vi "BoxSimShoot.vi"() -> ()   [LabVIEW 2023]
uses:
  BoxSystem/BoxStatesEnum.ctl
  BoxSystem/BoxNoteState.ctl
  <vilib>/Rock Robotics/WPI/ThirdParty/JAS_Junk/TrajLib/Enum/DCMOTOR_TYPES_ENUM.ctl
  <vilib>/Rock Robotics/WPI/ThirdParty/JAS_Junk/TrajLib/VI/Util_GetTime_U32.vi
  <vilib>/Rock Robotics/WPI/ThirdParty/JAS_Junk/TrajLib/VI/DigSeqLogic_Edge_On.vi
  <vilib>/Rock Robotics/WPI/ThirdParty/JAS_Junk/TrajLib/VI/BoolCmd_Send_Internal.vi
  <vilib>/Rock Robotics/WPI/ThirdParty/JAS_Junk/TrajLib/SlewRateLimiter_New.vi
  <vilib>/Rock Robotics/WPI/ThirdParty/JAS_Junk/TrajLib/SlewRateLimiter_Reset.vi
  <vilib>/Rock Robotics/WPI/ThirdParty/JAS_Junk/TrajLib/SlewRateLimiter_Calculate.vi
  <vilib>/Rock Robotics/WPI/ThirdParty/JAS_Junk/TrajLib/SlewRateLimiter_SetRate.vi
  <vilib>/Rock Robotics/WPI/ThirdParty/JAS_Junk/TrajLib/VI/BoolCmd_ObtainQueue.vi
  <vilib>/Rock Robotics/WPI/ThirdParty/JAS_Junk/TrajLib/VI/Util_GetTime_U64.vi
  <vilib>/Rock Robotics/WPI/ThirdParty/JAS_Junk/TrajLib/Trajectory_Library.lvlib
panel:
  out "Intake Control":T1(graph)
  in  "Cancel":bool
  in  "Amp":bool
  in  "Source":bool
  in  "Intake":bool
  in  "Shoot":bool
  out "Box Note State":T2
  out "StateMachineState":T3=enum."initilization"
  in  "Intake Sensor\nOff=BeamBroken":bool
  in  "Shoot Sensor\nOff=BeamBroken":bool
  out "Velocity_Filtered RPM R":dbl format="%13.1f"
  out "Velocity_Filtered RPM":dbl format="%13.1f"
  out "Motor DmdR (CO)":dbl format="%10.3f"
  out "AtSetpoint R":bool
  out "FeedForward R":dbl
  out "VelocityR_RPM":dbl format="%13.1f"
  in  "Auto R":bool=TRUE
  out "ShooterR Control":T4(graph)
  out "Battery Voltage":dbl format="%10.1f"
  out "ShooterL Control":T1(graph)
  in  "Auto":bool=TRUE
  out "VelocityL_RPM":dbl format="%13.1f"
  out "FeedForward":dbl
  out "AtSetpointL":bool
  out "MotorL Dmd (CO)":dbl format="%10.3f"
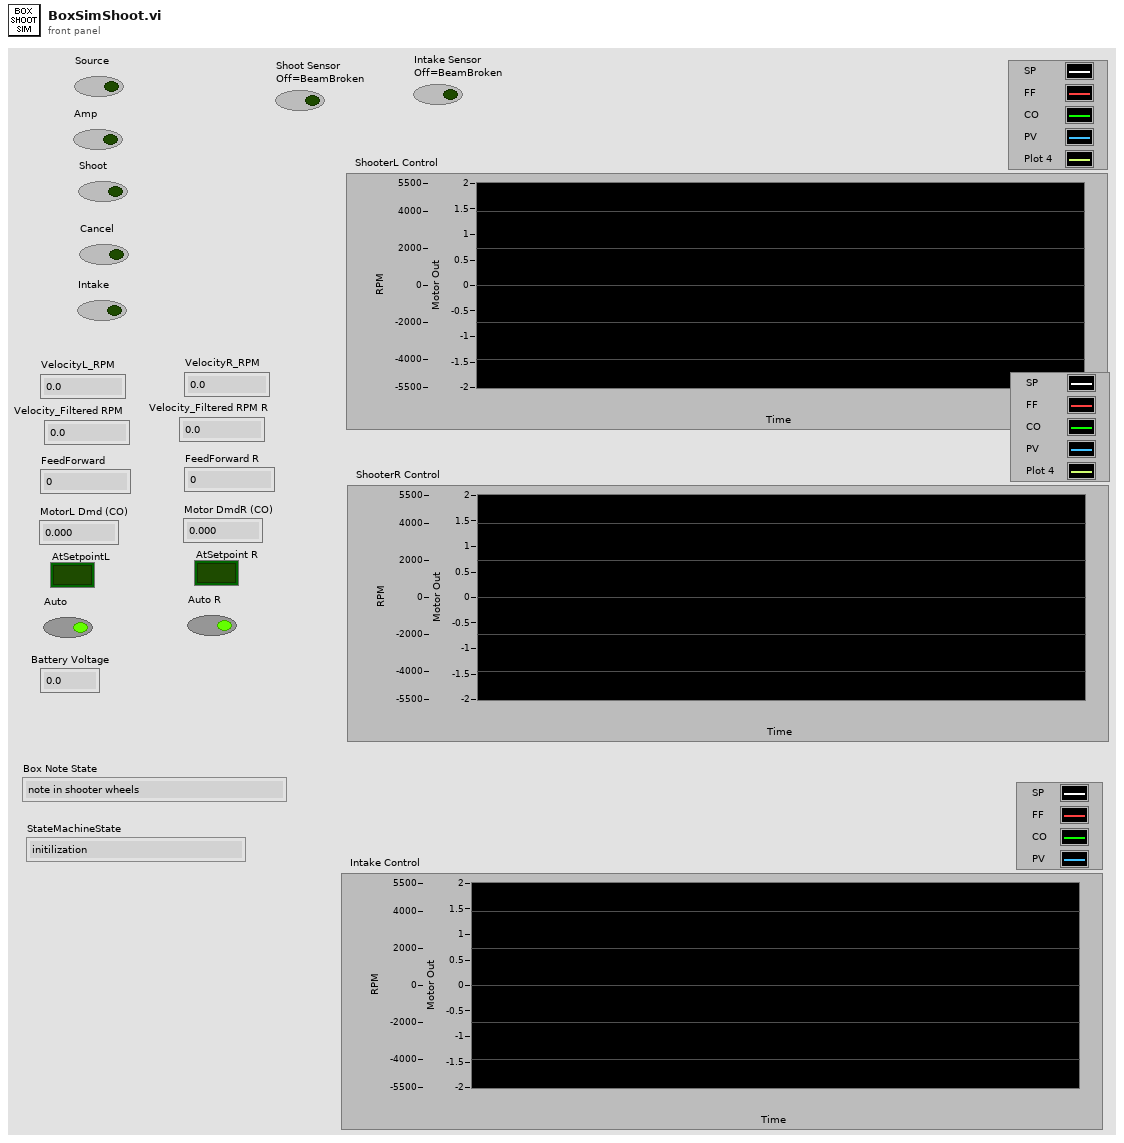
[diagram p1: front panel]
types:
  T1 = cluster{"ShootL SP":dbl, "ShootL FF":dbl, "ShootLOut":dbl, "Velocity_RPM":dbl, "ShootL Filt RPM":dbl}
  T2 = typedef "BoxNoteState.ctl" = enum16{"note in shooter wheels", "misaligned note", "no note", "have note"}
  T3 = typedef "BoxStatesEnum.ctl" = enum16{"get input", "start shoot wheels", "up to speed?", "run intake", "have ring?", "stop intake and shooter", "start intake", "pick up ring or  _ sec?", "stop intake", "start source  intake", "pick up note?", "stop intake shooter", "shoot amp", "used note?", "stop amp intake", "initilization"}
  T4 = cluster{"ShootR SP":dbl, "ShootR FF":dbl, "ShootROut":dbl, "Velocity_RPM":dbl, "ShootR Filt RPM":dbl}
  T5 = cluster{"Shoot Sensor":bool, "Intake Sensor":bool, "ShootLSpeed":dbl, "ShootRSpeed":dbl, "IntakeSpeed":dbl}
  T6 = typedef "Trajectory_Library.lvlib/DCMOTOR_TYPES_ENUM.ctl" = enum16{"CIM", "AndyMark 9015", "Andy Mark RS 775 125", "Bag", "BaneBots RS 550", "BaneBots RS 775", "Falcon 500", "Mini CIM", "NEO", "NEO 550", "Romi BuiltIn", "Vex 775 Pro", "Snow Blower AM 2235A", "Bosch Seat AM 3493"}
  T7 = cluster{"ShootLOnTarg":bool, "ShootROnTarg":bool, "StateMachineState":T3, "Box Note State":T2, "ShootR SP":dbl, "ShootR FF":dbl, "ShootR Filt RPM":dbl, "ShootL SP":dbl, "ShootL FF":dbl, "ShootL Filt RPM":dbl}
  T8 = cluster{"ShootLOut":dbl, "ShootROut":dbl, "IntakeOut":dbl}
  T9 = typedef "Trajectory_Library.lvlib/LINEAR_SYSTEM_ID_FLYWHEEL_MODEL.ctl" = cluster{"DCMOTOR_TYPES":T6, "Num Motors":i32, "Gearing":dbl, "MOI kgm2":dbl}
  T10 = typedef "Trajectory_Library.lvlib/FLYWHEEL_SIM_SIMULATION_PARAMS.ctl" = cluster{"Vel Meas Std Dev Rad/Sec":dbl}
  T11 = cluster{dbl, dbl, "IntakeOut":dbl, "Velocity_RPM":dbl, "Velocity_RPM":dbl}
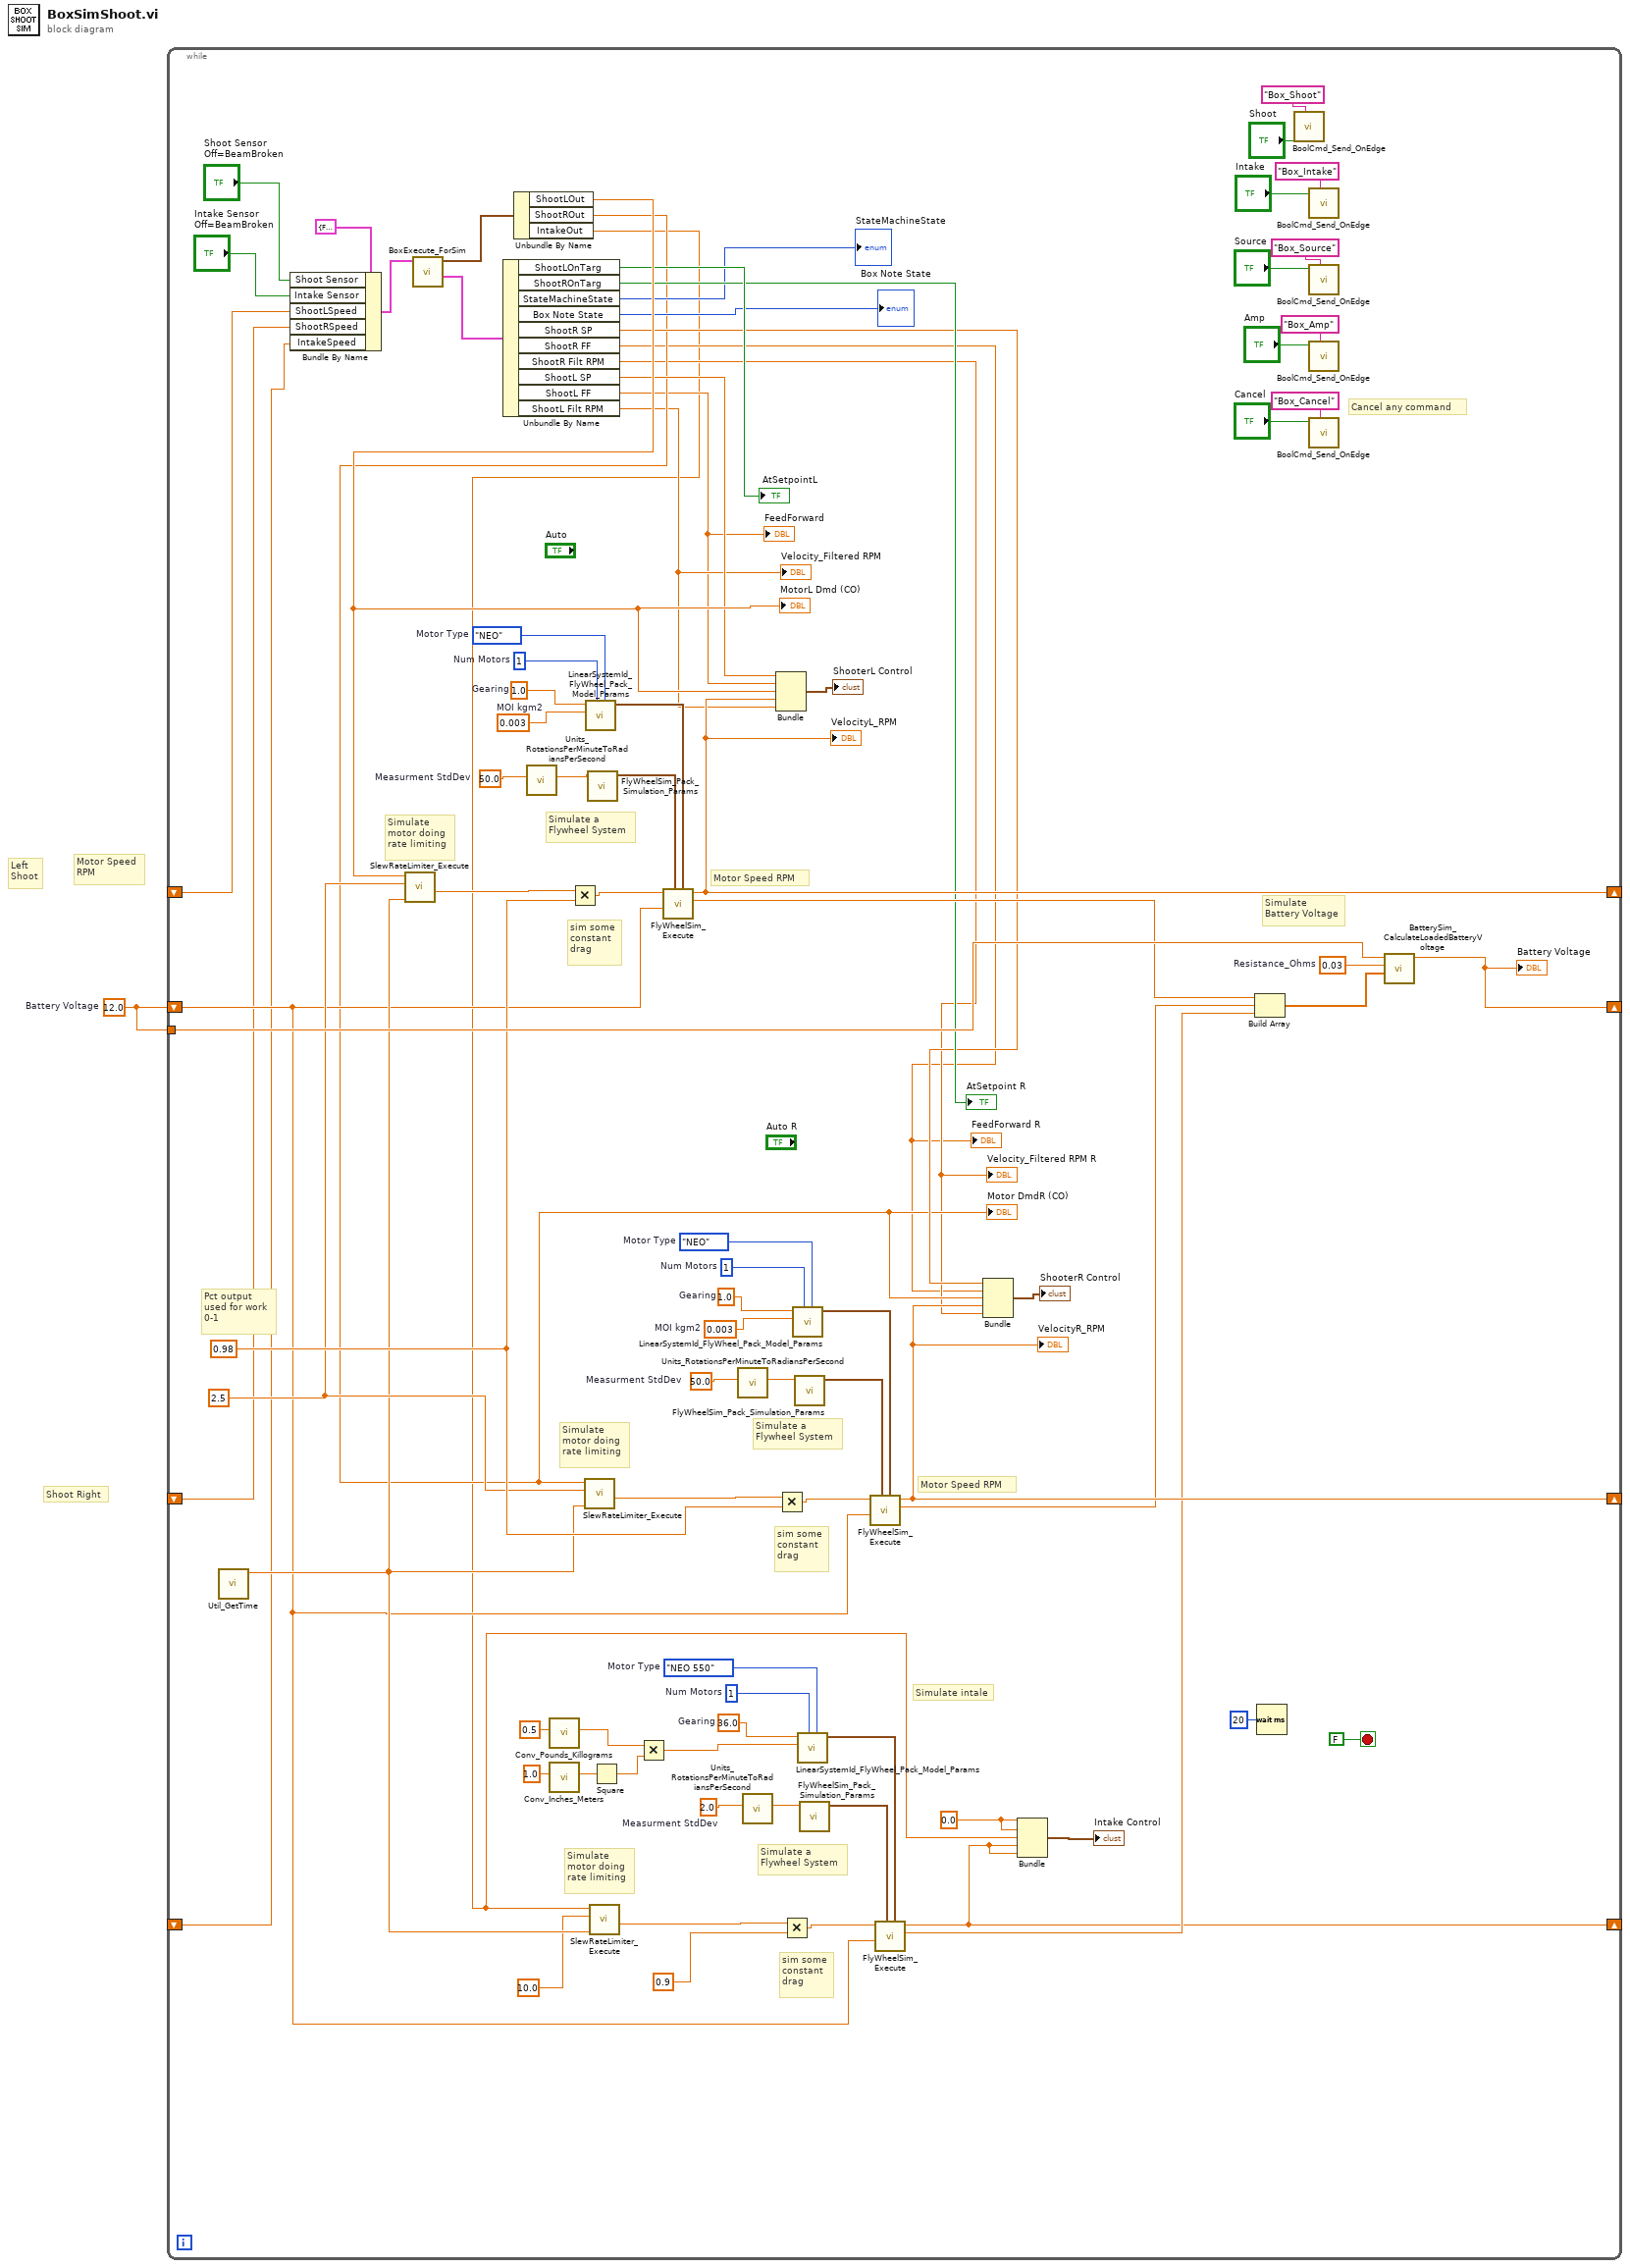
[diagram p0: block diagram]
diagram:
  w1 = 12.0  # Battery Voltage
  # "Shoot Right"
  # "Left\nShoot"
  # "Motor Speed\nRPM"
  n1 = while {
    shift-right: [w66] -> _
    shift-left: w1 -> [w38]
    shift-right: [w80] -> _
    shift-left: _ -> [w33]
    tunnel: w1 -> [w67]
    shift-right: [w69] -> _
    shift-left: _ -> [w32]
    shift-right: [w2] -> _
    shift-left: _ -> [w28]
    stop <- FALSE stop-if-true
    w4 = 0.0
    w48 = 2.0  # Measurment StdDev
    w50 = 36.0  # Gearing
    w51 = 1  # Num Motors
    w52 = DCMOTOR_TYPES_ENUM."NEO 550"  # Motor Type
    w58 = 50.0  # Measurment StdDev
    w61 = 2.5 ("y")
    w68 = 0.03  # Resistance_Ohms
    w59 = 50.0  # Measurment StdDev
    w70 = 1.0  # Gearing
    w71 = 0.003  # MOI kgm2
    w72 = 1  # Num Motors
    w73 = DCMOTOR_TYPES_ENUM."NEO"  # Motor Type
    w62 = 0.98 ("y")
    w87 = 1.0  # Gearing
    w88 = 0.003  # MOI kgm2
    w89 = 1  # Num Motors
    w90 = DCMOTOR_TYPES_ENUM."NEO"  # Motor Type
    # "Cancel any command"
    # "Simulate intale"
    # "Simulate\nmotor doing\nrate limiting"
    # "sim some\nconstant\ndrag"
    # "Simulate a \nFlywheel System"
    # "Pct output\nused for work\n0-1"
    # "Simulate\nmotor doing\nrate limiting"
    # "sim some\nconstant\ndrag"
    # "Motor Speed RPM"
    # "Simulate a \nFlywheel System"
    # "Simulate\nmotor doing\nrate limiting"
    # "sim some\nconstant\ndrag"
    # "Motor Speed RPM"
    # "Simulate\nBattery Voltage"
    # "Simulate a \nFlywheel System"
    n2 = call <vilib>:"Util_GetTime.vi"() -> ("FPGA_Time_Seconds"=w39:dbl)  [unwired: 9 in, 2 out]
    n3 = Bundle By Name(cluster=T5 {"Shoot Sensor"=FALSE, "Intake Sensor"=FALSE, "ShootLSpeed"=0.0, "ShootRSpeed"=0.0, "IntakeSpeed"=0.0} ("Inputs"), "Shoot Sensor"="Shoot Sensor\nOff=BeamBroken", "Intake Sensor"="Intake Sensor\nOff=BeamBroken", "ShootLSpeed"=w33, "ShootRSpeed"=w32, "IntakeSpeed"=w28) -> (w34:T5)
    n4 = call "BoxExecute_ForSim.vi"("Inputs"=w34) -> ("OtherOutputs"=w36:T7, "Outputs"=w37:T8)  [unwired: 9 in]
    n5 = Unbundle By Name(w36) -> ("ShootLOnTarg"=→"AtSetpointL":bool, "ShootROnTarg"=→"AtSetpoint R":bool, "StateMachineState"=→"StateMachineState":T3, "Box Note State"=→"Box Note State":T2, "ShootR SP"=w21:dbl, "ShootR FF"=w18:dbl, "ShootR Filt RPM"=w19:dbl, "ShootL SP"=w22:dbl, "ShootL FF"=w16:dbl, "ShootL Filt RPM"=w17:dbl)
    "FeedForward" <- w16
    "Velocity_Filtered RPM" <- w17
    "FeedForward R" <- w18
    "Velocity_Filtered RPM R" <- w19
    n6 = Unbundle By Name(w37) -> ("ShootLOut"=w31:dbl, "ShootROut"=w20:dbl, "IntakeOut"=w3:dbl)
    "MotorL Dmd (CO)" <- w31
    "Motor DmdR (CO)" <- w20
    n7 = call <vilib>:"SlewRateLimiter_Execute.vi"("Time"=w39, "PositiveRate"=w61, "Input"=w31) -> ("Output"=w79:dbl)  [unwired: 7 in, 1 out]
    n8 = call <vilib>:"Units_RotationsPerMinuteToRadiansPerSecond.vi"("RotationsPerMinute"=w58) -> ("RadiansPerSecond"=w57:dbl)  [unwired: 10 in]
    n9 = call <vilib>:"Conv_Pounds_Killograms.vi"("Pounds"=0.5) -> ("Killograms"=w45:dbl)  [unwired: 10 in]
    n10 = call <vilib>:"Conv_Inches_Meters.vi"("INCH"=1.0) -> ("Meters"=w47:dbl)  [unwired: 10 in]
    n11 = Multiply(x=w79, y=w62) -> (x*y=w82:dbl)
    n12 = call <vilib>:"SlewRateLimiter_Execute.vi"("Time"=w39, "PositiveRate"=w61, "Input"=w20) -> ("Output"=w78:dbl)  [unwired: 7 in, 1 out]
    n13 = call <vilib>:"LinearSystemId_FlyWheel_Pack_Model_Params.vi"("DCMOTOR_TYPES"=w90, "Num Motors"=w89, "MOI kgm2"=w88, "Gearing"=w87) -> ("LinearSystem_ID_FlyWheel_Model"=w84:T9)  [unwired: 7 in]
    n14 = call <vilib>:"FlyWheelSim_Pack_Simulation_Params.vi"("Vel Meas StdDev Rad/Sec"=w57) -> ("FlyWheelSim_Simulation_Params"=w83:T10)  [unwired: 10 in]
    n15 = call <vilib>:"SlewRateLimiter_Execute.vi"("Time"=w39, "PositiveRate"=10.0, "Input"=w3) -> ("Output"=w56:dbl)  [unwired: 7 in, 1 out]
    n16 = Square(x=w47) -> (x^2=w46:dbl)
    n17 = Multiply(x=w45, y=w46) -> (x*y=w42:dbl)
    n18 = call <vilib>:"FlyWheelSim_Execute.vi"("FlyWheelSim_Model _Params"=w84, "FlyWheelSim_Simulation_Params"=w83, "Battery Volts"=w38, "Motor Dmd"=w82) -> ("Motor Current"=w65:dbl, "Velocity_RPM"=w80:dbl)  [unwired: 4 in, 2 out]
    "VelocityL_RPM" <- w80
    n19 = call <vilib>:"Units_RotationsPerMinuteToRadiansPerSecond.vi"("RotationsPerMinute"=w59) -> ("RadiansPerSecond"=w60:dbl)  [unwired: 10 in]
    n20 = call <vilib>:"Units_RotationsPerMinuteToRadiansPerSecond.vi"("RotationsPerMinute"=w48) -> ("RadiansPerSecond"=w49:dbl)  [unwired: 10 in]
    n21 = Bundle("ShootL SP"=w22, "ShootL FF"=w16, "ShootLOut"=w31, "Velocity_RPM"=w80, "ShootL Filt RPM"=w17) -> (→"ShooterL Control":T1)  [unwired: 1 in]
    n22 = Multiply(x=w78, y=w62) -> (x*y=w76:dbl)
    n23 = Multiply(x=w56, y=0.9) -> (x*y=w55:dbl)
    n24 = call <vilib>:"LinearSystemId_FlyWheel_Pack_Model_Params.vi"("DCMOTOR_TYPES"=w73, "Num Motors"=w72, "MOI kgm2"=w71, "Gearing"=w70) -> ("LinearSystem_ID_FlyWheel_Model"=w74:T9)  [unwired: 7 in]
    n25 = call <vilib>:"FlyWheelSim_Pack_Simulation_Params.vi"("Vel Meas StdDev Rad/Sec"=w60) -> ("FlyWheelSim_Simulation_Params"=w75:T10)  [unwired: 10 in]
    n26 = call <vilib>:"LinearSystemId_FlyWheel_Pack_Model_Params.vi"("DCMOTOR_TYPES"=w52, "Num Motors"=w51, "MOI kgm2"=w42, "Gearing"=w50) -> ("LinearSystem_ID_FlyWheel_Model"=w53:T9)  [unwired: 7 in]
    n27 = call <vilib>:"FlyWheelSim_Pack_Simulation_Params.vi"("Vel Meas StdDev Rad/Sec"=w49) -> ("FlyWheelSim_Simulation_Params"=w54:T10)  [unwired: 10 in]
    n28 = call <vilib>:"FlyWheelSim_Execute.vi"("FlyWheelSim_Model _Params"=w74, "FlyWheelSim_Simulation_Params"=w75, "Battery Volts"=w38, "Motor Dmd"=w76) -> ("Motor Current"=w64:dbl, "Velocity_RPM"=w69:dbl)  [unwired: 4 in, 2 out]
    "VelocityR_RPM" <- w69
    n29 = call <vilib>:"FlyWheelSim_Execute.vi"("FlyWheelSim_Model _Params"=w53, "FlyWheelSim_Simulation_Params"=w54, "Battery Volts"=w38, "Motor Dmd"=w55) -> ("Motor Current"=w40:dbl, "Velocity_RPM"=w2:dbl)  [unwired: 4 in, 2 out]
    n30 = Bundle("ShootR SP"=w21, "ShootR FF"=w18, "ShootROut"=w20, "Velocity_RPM"=w69, "ShootR Filt RPM"=w19) -> (→"ShooterR Control":T4)  [unwired: 1 in]
    n31 = Bundle(w4, w4, "IntakeOut"=w3, "Velocity_RPM"=w2, "Velocity_RPM"=w2) -> (→"Intake Control":T11)  [unwired: 1 in]
    n32 = Build Array(w65, w64, w40) -> (w63:dbl[])
    n33 = Wait (ms)(milliseconds to wait=u32 20) -> ()  [unwired: 1 out]
    n34 = call <vilib>:"BoolCmd_Send_OnEdge.vi"("Command Name"="Box_Shoot", "Value"="Shoot") -> ()  [unwired: 9 in, 1 out]
    n35 = call <vilib>:"BoolCmd_Send_OnEdge.vi"("Command Name"="Box_Intake", "Value"="Intake") -> ()  [unwired: 9 in, 1 out]
    n36 = call <vilib>:"BoolCmd_Send_OnEdge.vi"("Command Name"="Box_Source", "Value"="Source") -> ()  [unwired: 9 in, 1 out]
    n37 = call <vilib>:"BoolCmd_Send_OnEdge.vi"("Command Name"="Box_Amp", "Value"="Amp") -> ()  [unwired: 9 in, 1 out]
    n38 = call <vilib>:"BoolCmd_Send_OnEdge.vi"("Command Name"="Box_Cancel", "Value"="Cancel") -> ()  [unwired: 9 in, 1 out]
    n39 = call <vilib>:"BatterySim_CalculateLoadedBatteryVoltage.vi"("Currents"=w63, "Resistance_Ohms"=w68, "NominalVoltage"=w67) -> ("Voltage"=w66:dbl)  [unwired: 8 in]
    "Battery Voltage" <- w66
  }
